vi "Lab0_Case.vi"() -> ()   [LabVIEW 2014]
panel:
  in  "stop":bool
  out "String":string
  in  "Boolean":bool
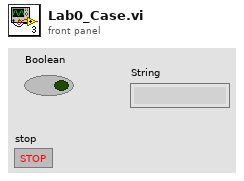
[diagram p1: front panel]
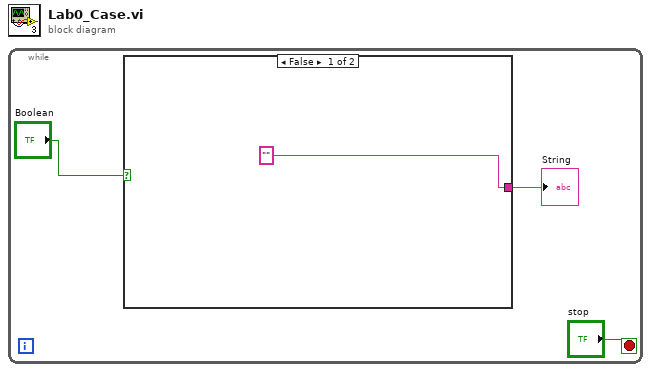
[diagram p0: block diagram]
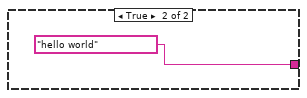
[diagram p2: hidden frame]
diagram:
  n1 = while {
    stop <- "stop" stop-if-true
    n2 = case shown="False" "Boolean" {
      tunnel: ["" "hello world"] -> w1
      frame False {
      }
      frame True {
      }
    }
    "String" <- w1
  }
